vi "sutter_test.vi"() -> ()   [LabVIEW 2016]
uses:
  <vilib>/Instr/_visa.llb/VISA Configure Serial Port (Instr).vi
panel:
  in  "Manipulator":u16(ring) items=["DriveA"=1, "DriveB"=2]
  in  "Motor Position":dbl[](array[numeric])
  out "Position XYZ":dbl[](array[numeric])
  in  "Ring":u16(ring) items=["Move to work", "Move to home", "Calibration", "Get pos", "Interrupt", "Move to pos", "ChangeDrive"]
  in  "error in (no error)":errorcluster
  out "error out":errorcluster
  in  "VISA resource name":refnum<visa-resource-name>
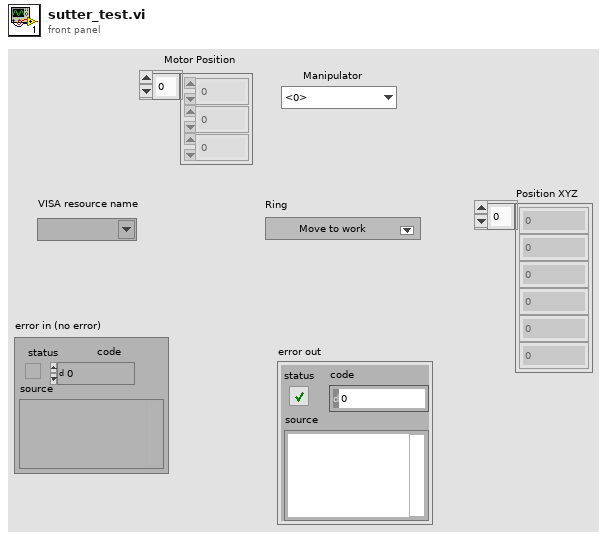
[diagram p1: front panel]
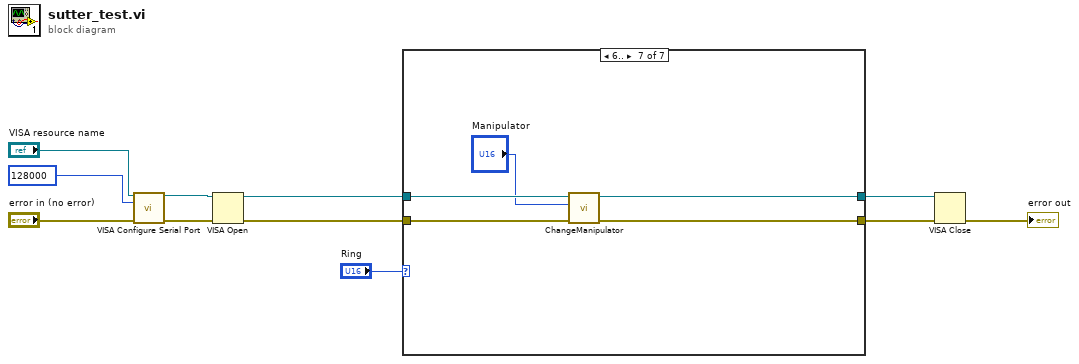
[diagram p0: block diagram]
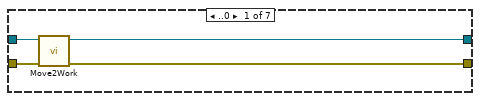
[diagram p2: hidden frame]
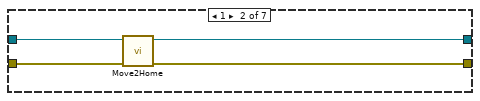
[diagram p3: hidden frame]
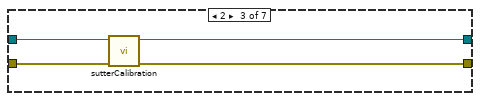
[diagram p4: hidden frame]
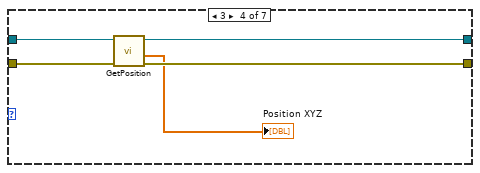
[diagram p5: hidden frame]
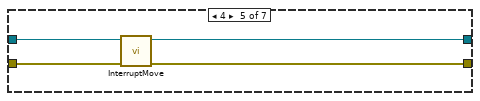
[diagram p6: hidden frame]
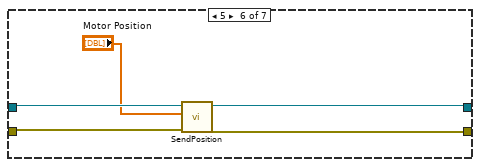
[diagram p7: hidden frame]
diagram:
  n1 = call-poly "VISA Configure Serial Port"("VISA resource name"="VISA resource name", "baud rate (9600)"=u32 128000, "error in (no error)"="error in (no error)") -> ("VISA resource name out"=w8:refnum<visa-resource-name>, "error out"=w6:errorcluster)  [unwired: 11 in]
  n2 = VISA Open(error in (no error)=w6, VISA resource name=w8) -> (VISA resource name=w5:refnum<visa-resource-name>, error out=w4:errorcluster)  [unwired: 3 in]
  n3 = case shown="6.." "Ring" {
    tunnel: w5 -> [w15 w18 w23 w28 w32 w37 w42]
    tunnel: w4 -> [w14 w19 w22 w26 w31 w36 w41]
    tunnel: [w13 w16 w20 w25 w29 w34 w39] -> w3
    tunnel: [w12 w17 w21 w27 w30 w35 w40] -> w2
    frame ..0 {
      n4 = call "Move2Work.vi"("error in"=w14, "VISA resource In"=w15) -> ("error out"=w13:errorcluster, "VISA resource name out"=w12:refnum<visa-resource-name>)  [unwired: 6 in]
    }
    frame 1 {
      n5 = call "Move2Home.vi"("error in"=w19, "VISA resource In"=w18) -> ("error out"=w16:errorcluster, "VISA resource name out"=w17:refnum<visa-resource-name>)  [unwired: 6 in]
    }
    frame 2 {
      n6 = call "sutterCalibration.vi"("error in"=w22, "VISA resource In"=w23) -> ("error out"=w20:errorcluster, "VISA resource name out"=w21:refnum<visa-resource-name>)  [unwired: 6 in]
    }
    frame 3 {
      n7 = call "GetPosition.vi"("error in"=w26, "VISA resource name in"=w28) -> ("error out"=w25:errorcluster, "Position XYZ"=→"Position XYZ":dbl[], "VISA resource name out"=w27:refnum<visa-resource-name>)  [unwired: 3 in, 1 out]
    }
    frame 4 {
      n8 = call "InterruptMove.vi"("error in"=w31, "VISA resource In"=w32) -> ("error out"=w29:errorcluster, "VISA resource name out"=w30:refnum<visa-resource-name>)  [unwired: 6 in]
    }
    frame 5 {
      n9 = call "SendPosition.vi"("error in"=w36, "Motor Position"="Motor Position", "VISA resource In"=w37) -> ("error out"=w34:errorcluster, "VISA resource name out"=w35:refnum<visa-resource-name>)  [unwired: 5 in]
    }
    frame 6.. {
      n10 = call "ChangeManipulator.vi"("error in"=w41, "Manipulator"="Manipulator", "VISA resource In"=w42) -> ("error out"=w39:errorcluster, "VISA resource name out"=w40:refnum<visa-resource-name>)  [unwired: 5 in]
    }
  }
  n11 = VISA Close(VISA resource name=w2, error in (no error)=w3) -> (error out=→"error out":errorcluster)
